vi "Read Test Parameters.vi"(11 "TestMonitor in":refnum<class "TestMonitor.lvclass">) -> (2 "Test Parameters":T1={"Number of cycles for complete test"=0, "Cycle profile"={"Temperature Setpoint"=[], "Soak Time"=[], "Gain Stabilization Time"=[], "Pause After Step"=[]}, "PGA Gain Coefficients"=[], "Temperature Transition Wait Time"=0.0, "Temperature Settled StDev"=273.15, "Temperature Settling Sample Size"=0, "Bridge Measurement Sample Size"=0} {"Temperature Settling Sample Size" min=1; "Bridge Measurement Sample Size" min=1; "Temperature Settled StDev" min=271.15 max=275.15 format="%.4f"; "PGA Gain Coefficients" max=7; "Temperature Transition Wait Time" min=1.0; "Cycle profile"."Gain Stabilization Time" min=0.0 max=600.0 format="%.1f"; "Cycle profile"."Soak Time" min=0.0 max=600.0 format="%.1f"; "Cycle profile"."Pause After Step" min=0.0 max=600.0 format="%.1f"; "Cycle profile"."Temperature Setpoint" min=233.14999999999998 max=313.15 format="%.1f"; "Number of cycles for complete test" min=1}, 3 "TestMonitor out":refnum<class "TestMonitor.lvclass">)   [LabVIEW 2013, in "TestMonitor.lvclass"]
uses:
  TestMonitor.lvclass
  Configuration/TestParameters.ctl
  Configuration/CycleProfileConfig.ctl
  TestMonitor.lvclass/TestMonitor.ctl
panel:
  # "Gain is 2^gain_coefficient"
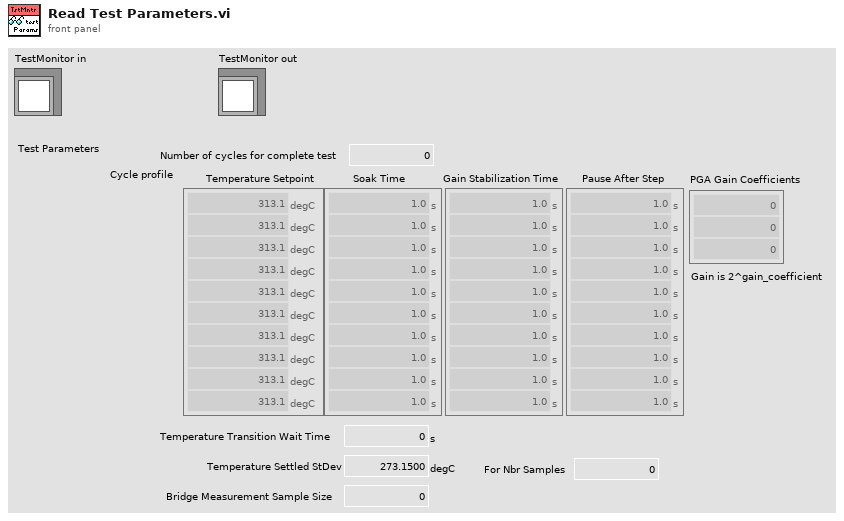
[diagram p1: front panel]
types:
  T1 = typedef "TestParameters.ctl" = cluster{"Number of cycles for complete test":u32, "Cycle profile":T2, "PGA Gain Coefficients":u8[], "Temperature Transition Wait Time":dbl[unit], "Temperature Settled StDev":dbl[unit], "Temperature Settling Sample Size":u16, "Bridge Measurement Sample Size":u16}
  T2 = typedef "CycleProfileConfig.ctl" = cluster{"Temperature Setpoint":dbl[unit][], "Soak Time":dbl[unit][], "Gain Stabilization Time":dbl[unit][], "Pause After Step":dbl[unit][]}
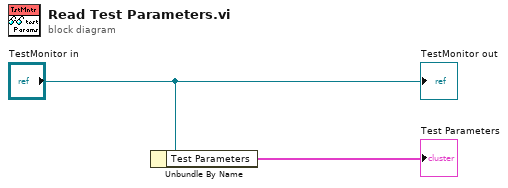
[diagram p0: block diagram]
diagram:
  n1 = Unbundle By Name("TestMonitor in") -> ("Test Parameters"=→"Test Parameters":T1)
  "TestMonitor out" <- "TestMonitor in"
